vi "Write to Log.vi"(8 "error in (no error)":errorcluster, 10 "Text to Write":string, 11 "Log in":refnum<class "Log Mock.lvclass">) -> (0 "error out":errorcluster, 3 "Log out":refnum<class "Log Mock.lvclass">)   [LabVIEW 2020, in "Log Mock.lvclass"]
uses:
  Log Mock.lvclass
  C:/Program Files (x86)/National Instruments/LabVIEW 2020/vi.lib/Astemes/LMock/Mock.lvclass
  <vilib>/Astemes/LMock/Mock.lvclass
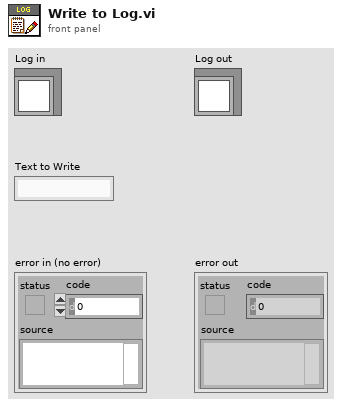
[diagram p1: front panel]
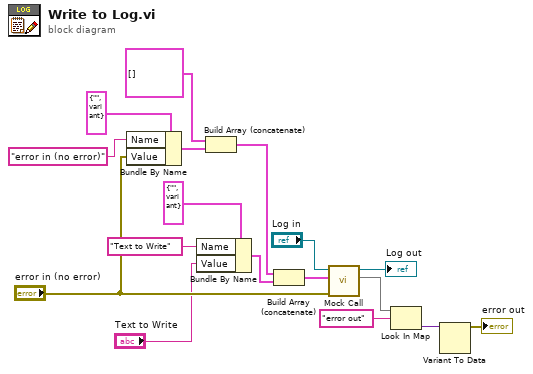
[diagram p0: block diagram]
diagram:
  n1 = Bundle By Name(cluster=cluster{"Name":string, "Value":variant} {"Name"="", "Value"=variant} ("element"), "Name"="error in (no error)", "Value"="error in (no error)") -> (w3:cluster{"Name":string, "Value":variant})
  n2 = Bundle By Name(cluster=cluster{"Name":string, "Value":variant} {"Name"="", "Value"=variant} ("element"), "Name"="Text to Write", "Value"="Text to Write") -> (w1:cluster{"Name":string, "Value":variant})
  n3 = Build Array (concatenate)(cluster{"Name":string, "Value":variant}[] [] ("Control Values"), w3) -> (w11:cluster{"Name":string, "Value":variant}[])
  n4 = Build Array (concatenate)(w11, w1) -> (w14:cluster{"Name":string, "Value":variant}[])
  n5 = call <vilib>:"Mock Call.vi"("error in (no error)"="error in (no error)", "Control Values"=w14, "Mock In"="Log in") -> ("Input Parameters"=w9:map{string, variant}, "Mock Out"=→"Log out":refnum<class "Log Mock.lvclass">)  [unwired: 7 in]
  n6 = Look In Map(map=w9, key="error out") -> (value=w7:variant)  [unwired: 1 in, 1 out]
  n7 = Variant To Data(Variant=w7) -> (data=→"error out":errorcluster)  [unwired: 2 in, 1 out]
